vi "Subvi PMT simulator.vi"(9 "Pulse sequence":bool[](array[boolean])=[FALSE, FALSE, FALSE, FALSE, FALSE, FALSE, FALSE, FALSE, FALSE, FALSE]) -> ()   [LabVIEW 2017]
uses:
  <vilib>/rvi/eio/common/nirviEmuTemplateMethod_errors.vi
  <vilib>/eio/EIONode/EIONode.xnode
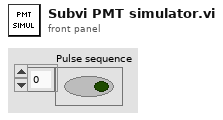
[diagram p1: front panel]
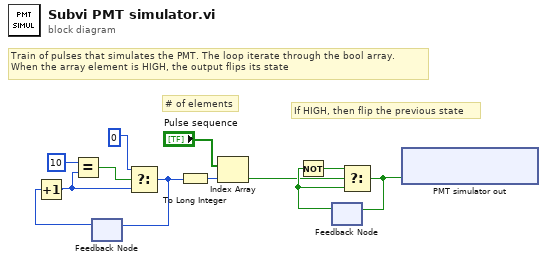
[diagram p0: block diagram]
diagram:
  # "If HIGH, then flip the previous state"
  # "# of elements"
  # "Train of pulses that simulates the PMT. The loop iterate through the bool array.\nWhen the array element is HIGH, the output flips its state"
  n1 = feedback #1() -> (w1:u8)  [unwired: 1 in]
  n2 = Increment(x=w1) -> (x+1=w2:u8)
  n3 = Equal?(x=u8 10, y=w2) -> (x = y?=w5:bool)
  n4 = Select(t=u8 0, s=w5, f=w2) -> (s? t:f=w3:u8)
  n5 = feedback-in #1(w3) -> ()
  n6 = To Long Integer(number=w3) -> (32bit integer=w4:i32)
  n7 = Index Array(array="Pulse sequence", index=w4) -> (element=w9:bool)
  n8 = feedback #2() -> (w11:bool)  [unwired: 1 in]
  n9 = Not(x=w11) -> (.not. x?=w10:bool)
  n10 = Select(t=w10, s=w9, f=w11) -> (s? t:f=w12:bool)
  n11 = feedback-in #2(w12) -> ()
  n12 = xnode "PMT simulator out"("Connector0/DIO1"=w12) -> ()  [unwired: 1 in, 1 out]
